vi "Get_Scaler_Rate.vi"(5 "Delay Time (s)":sgl=1.0) -> (0 "Duty Factor":dbl, 1 "Cluster out":T1)   [LabVIEW 2014]
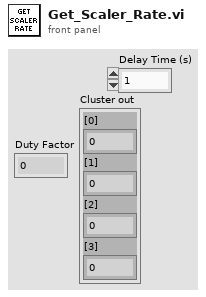
[diagram p1: front panel]
types:
  T1 = cluster{"[0]":dbl, "[1]":dbl, "[2]":dbl, "[3]":dbl}
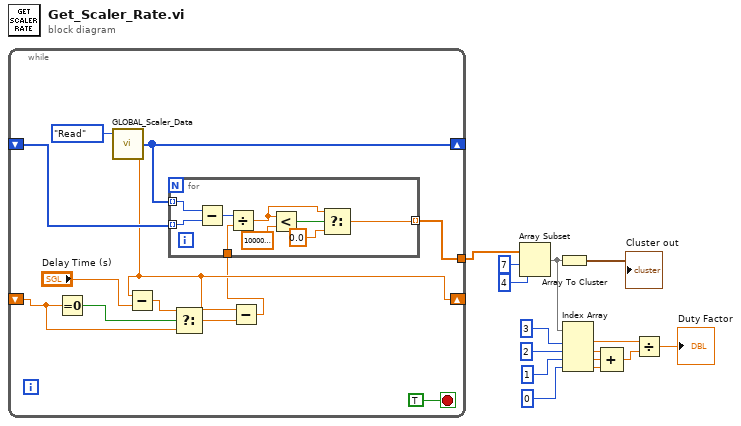
[diagram p0: block diagram]
diagram:
  n1 = while {
    shift-right: [w26] -> _
    shift-left: _ -> [w23]
    tunnel: [w24] -> w13
    shift-right: [w17] -> _
    shift-left: _ -> [w18]
    stop <- TRUE stop-if-true
    n2 = Equal To 0?(x=w18) -> (x = 0?=w22:bool)
    n3 = call "GLOBAL_Scaler_Data.vi"("State"=enum16{"Initialise", "Write", "Read"}."Read") -> ("Acquisition Time"=w17:dbl, "Data Out"=w26:u32[])  [unwired: 3 in]
    n4 = Subtract(x=w17, y="Delay Time (s)") -> (x-y=w20:dbl)
    n5 = Select(t=w20, s=w22, f=w18) -> (s? t:f=w21:dbl)
    n6 = Subtract(x=w17, y=w21) -> (x-y=w16:dbl)
    n7 = for {
      tunnel: w26 -> [w36] mode=indexing
      tunnel: w23 -> [w35] mode=indexing
      tunnel: [w29] -> w24 mode=indexing
      tunnel: w16 -> [w28]
      n8 = Subtract(x=w36, y=w35) -> (x-y=w34:u32)
      n9 = Divide(x=w34, y=w28) -> (x/y=w30:dbl)
      n10 = Less?(x=w30, y=sgl 1000000.0) -> (x < y?=w32:bool)
      n11 = Select(t=w30, s=w32, f=0.0) -> (s? t:f=w29:dbl)
    }
  }
  n12 = Array Subset(array=w13, index=7, length=4) -> (w11:dbl[])
  n13 = Array To Cluster(array=w11) -> (cluster=→"Cluster out":T1)
  n14 = Index Array(array=w11, index #1=3 ("index"), index #2=2 ("index"), index #3=1 ("index"), index #4=0 ("index")) -> (element #1=w9:dbl, element #2=w4:dbl, element #3=w3:dbl, element #4=w2:dbl)
  n15 = Compound Arithmetic op=ADD(w4, w3, w2) -> (w1:dbl)
  n16 = Divide(x=w9, y=w1) -> (x/y=→"Duty Factor":dbl)
